vi "ex3-5.vi"() -> ()   [LabVIEW 2009]
panel:
  in  "結束":bool
  out "Sine 波形圖":dbl(graph)
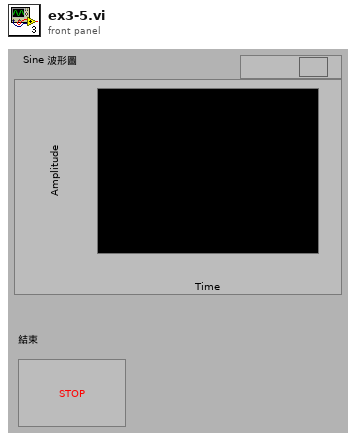
[diagram p1: front panel]
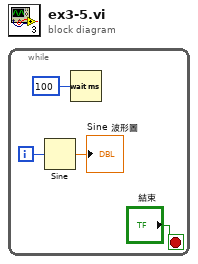
[diagram p0: block diagram]
diagram:
  n1 = while {
    i -> [w4]
    stop <- "結束" stop-if-true
    n2 = Sine(x=w4) -> (sin(x)=→"Sine 波形圖":dbl)
    n3 = Wait (ms)(milliseconds to wait=u32 100) -> ()  [unwired: 1 out]
  }
